vi "打开文件夹.vi"(8 "错误输入":errorcluster, 11 "文件夹":path) -> (0 "error out":errorcluster caption="错误输出")   [LabVIEW 2018]
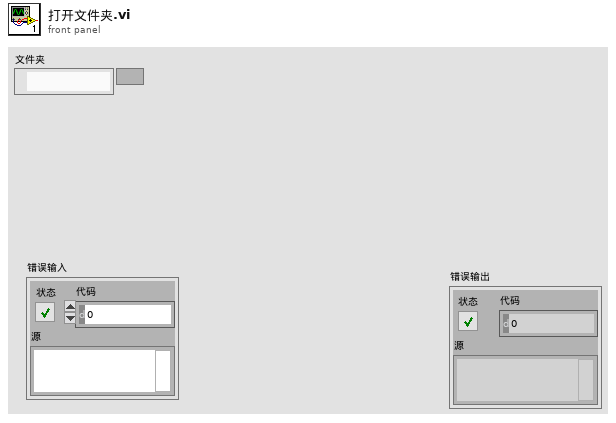
[diagram p1: front panel]
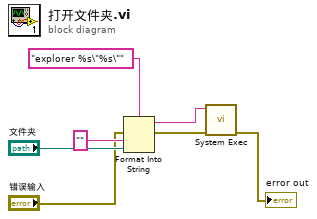
[diagram p0: block diagram]
diagram:
  n1 = Format Into String(format string="explorer %s\"%s\"", error in="错误输入", "" ("输入 1"), "文件夹") -> (resulting string=w5:string, error out=w4:errorcluster)  [unwired: 1 in]
  n2 = call <vilib>:"System Exec.vi"("error in (no error)"=w4, "command line"=w5) -> ("error out"=→"error out":errorcluster)  [unwired: 6 in, 3 out]
